vi "MGlogging.vi"(9 "New square":T1, 11 "Refnum in":refnum<k33>) -> (3 "tiggerTime":u32)   [LabVIEW 2020]
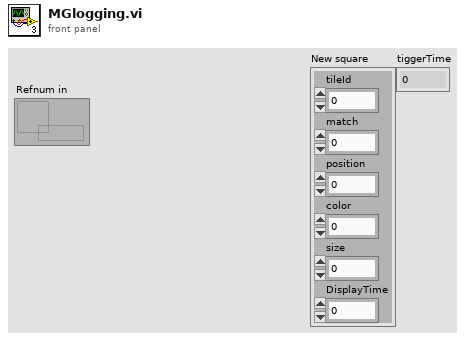
[diagram p1: front panel]
types:
  T1 = cluster{"tileId":i32, "match":i32, "position":i32, "color":u32, "size":i32, "DisplayTime":i32}
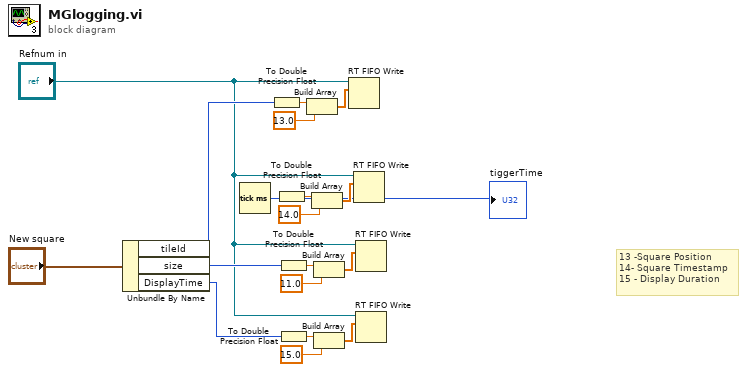
[diagram p0: block diagram]
diagram:
  # "13 -Square Position \n14- Square Timestamp\n15 - Display Duration"
  n1 = Unbundle By Name("New square") -> ("tileId"=w15:i32, "size"=w7:i32, "DisplayTime"=w1:i32)
  n2 = Tick Count (ms)() -> (millisecond timer value=w11:u32)
  "tiggerTime" <- w11
  n3 = To Double Precision Float(number=w15) -> (double precision float=w16:dbl)
  n4 = To Double Precision Float(number=w11) -> (double precision float=w13:dbl)
  n5 = To Double Precision Float(number=w7) -> (double precision float=w9:dbl)
  n6 = To Double Precision Float(number=w1) -> (double precision float=w5:dbl)
  n7 = Build Array(w16, 13.0 ("element")) -> (w18:dbl[])
  n8 = Build Array(w13, 14.0 ("element")) -> (w12:dbl[])
  n9 = Build Array(w9, 11.0 ("element")) -> (w8:dbl[])
  n10 = Build Array(w5, 15.0 ("element")) -> (w4:dbl[])
  n11 = RT FIFO Write(0:"Refnum in", 1:w18) -> ()  [unwired: 3 in, 4 out]
  n12 = RT FIFO Write(0:"Refnum in", 1:w12) -> ()  [unwired: 3 in, 4 out]
  n13 = RT FIFO Write(0:"Refnum in", 1:w8) -> ()  [unwired: 3 in, 4 out]
  n14 = RT FIFO Write(0:"Refnum in", 1:w4) -> ()  [unwired: 3 in, 4 out]
